vi "VIQA VI Info.vi"(8 "error in (no error)":errorcluster, 10 "Item ID":string, 11 "Project":refnum<vi>) -> (0 "error out":errorcluster, 1 "Valid?":bool, 2 "VI Info":T1, 3 "VI Refnum":refnum<vi>)   [LabVIEW 2018, in "VI Quality.lvlib"]
doc: "This returns VI information about the project item selected."
uses:
  VI Quality.lvlib
  <vilib>/LabVIEW Icon API/LabVIEW Icon API.lvlib
  <vilib>/LabVIEW Icon API/lv_icon/Classes/Icon/Icon.lvclass
  Controls/VIQA VI Info.ctl
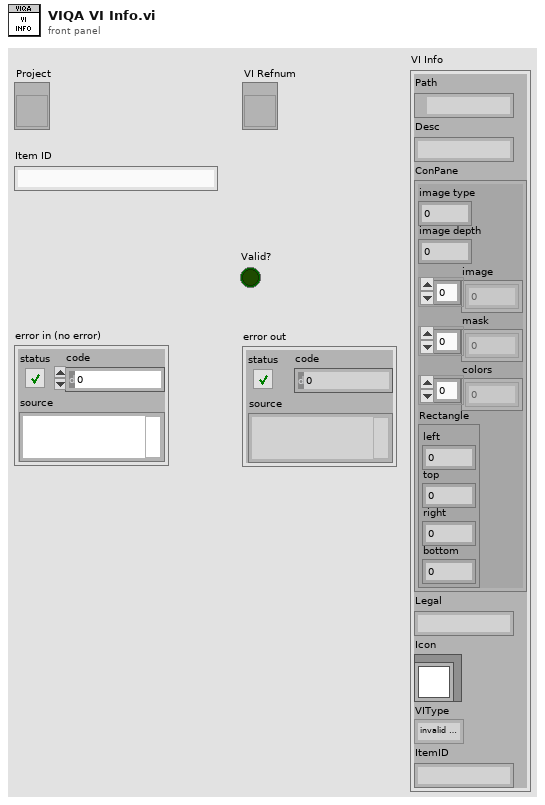
[diagram p1: front panel]
types:
  T1 = typedef "VI Quality.lvlib/VIQA VI Info.ctl" = cluster{"Path":path, "Desc":string, "ConPane":cluster{"image type":i32, "image depth":i32, "image":u8[], "mask":u8[], "colors":u32[], "Rectangle":cluster{"left":i16, "top":i16, "right":i16, "bottom":i16}}, "Legal":string, "Icon":refnum<class "Icon.lvclass">, "VIType":enum32{"invalid VI type", "Standard VI", "Control VI", "Global VI", "Polymorphic VI", "Configuration VI", "SubSystem", "Facade VI", "Method VI", "Statechart Diagram VI"}, "ItemID":string}
  T2 = enum32{"invalid VI type", "Standard VI", "Control VI", "Global VI", "Polymorphic VI", "Configuration VI", "SubSystem", "Facade VI", "Method VI", "Statechart Diagram VI"}
  T3 = typedef "imagedata.ctl" = cluster{"image type":i32, "image depth":i32, "image":u8[], "mask":u8[], "colors":u32[], "Rectangle":cluster{"left":i16, "top":i16, "right":i16, "bottom":i16}}
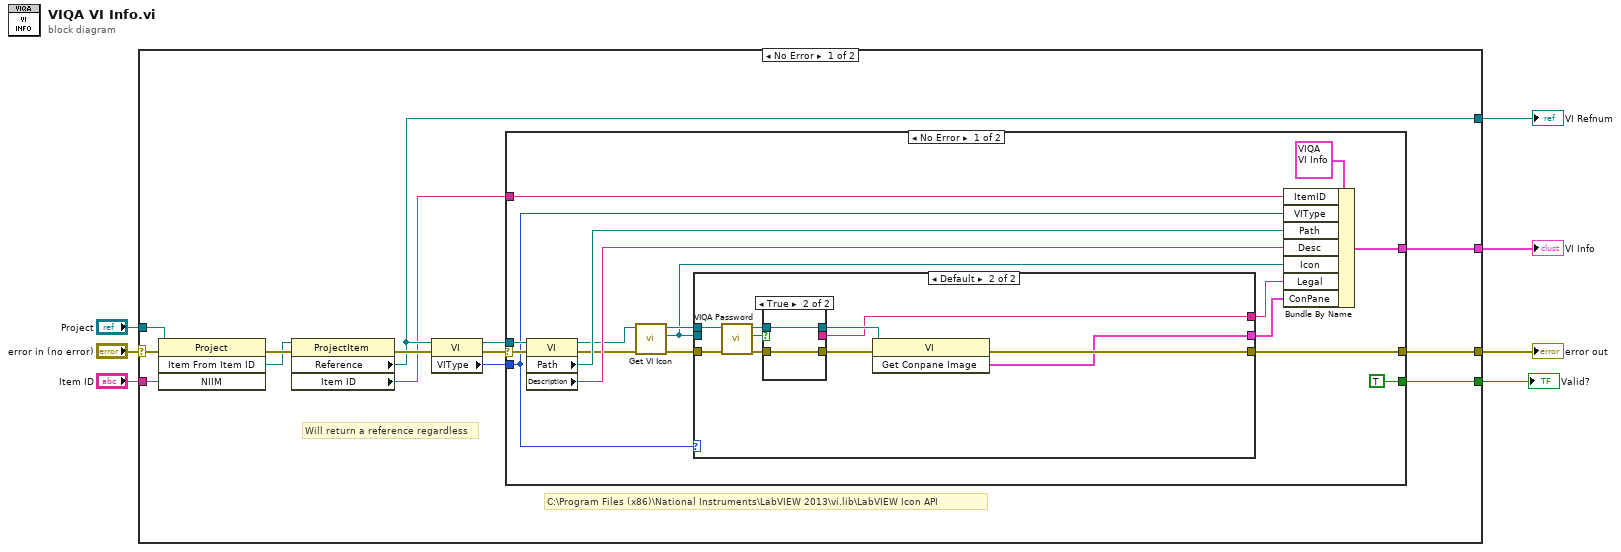
[diagram p0: block diagram]
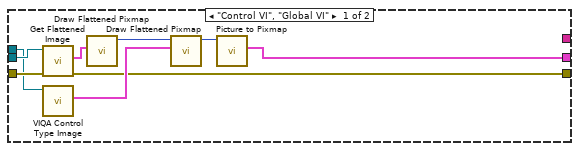
[diagram p2: hidden frame]
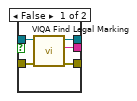
[diagram p3: hidden frame]
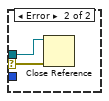
[diagram p4: hidden frame]
diagram:
  n1 = case shown="No Error" "error in (no error)" {
    selector: "error in (no error)" -> [w19 w67]
    tunnel: "Item ID" -> [w18 _]
    tunnel: "Project" -> [w17 _]
    tunnel: [w15 w67] -> w4
    tunnel: [w14 _] -> w3
    tunnel: [w13 _] -> w2
    tunnel: [w9 _] -> w1
    frame No Error {
      # "C:\\Program Files (x86)\\National Instruments\\LabVIEW 2013\\vi.lib\\LabVIEW Icon API"
      # "Will return a reference regardless"
      n2 = invoke class="Project" method="Item From Item ID"(reference=w17, error in=w19, "NIIM"=w18) -> (error out=w21:errorcluster, "GetItemFromNIIM"=w20:refnum<vi>)  [unwired: 1 in, 2 out]
      n3 = property class="ProjectItem"(reference=w20, error in=w21) -> (error out=w16:errorcluster, "Reference"=w13:refnum<vi>, "Item ID"=w8:string)  [unwired: 1 out]
      n4 = property class="VI"(reference=w13, error in=w16) -> (reference out=w12:refnum<vi>, error out=w11:errorcluster, "VIType"=w10:T2)
      n5 = case shown="No Error" w11 {
        selector: w11 -> [w32 w66]
        tunnel: [w38 _] -> w15
        tunnel: [w37 _] -> w14
        tunnel: w12 -> [w33 w65]
        tunnel: w10 -> [w23 _]
        tunnel: [TRUE _] -> w9
        tunnel: w8 -> [w22 _]
        frame No Error {
          n6 = property class="VI"(reference=w33, error in=w32) -> (reference out=w26:refnum<vi>, error out=w31:errorcluster, "Path"=w36:path, "Description"=w35:string)
          n7 = call <vilib>:"Get VI Icon.vi"("error in (no error)"=w31, "VI Refnum in"=w26) -> ("error out"=w30:errorcluster, "Icon"=w28:refnum<class "Icon.lvclass">, "VI Refnum out"=w29:refnum<vi>)  [unwired: 7 in]
          n8 = case shown="Default" w23 {
            tunnel: [w41 w57] -> w38
            tunnel: w30 -> [w47 w52]
            tunnel: w29 -> [w45 w50]
            tunnel: [w39 w56] -> w34
            tunnel: w28 -> [w46 _]
            tunnel: [_ w53] -> w24
            frame "Control VI", "Global VI" {
              n9 = call <vilib>:"Get Flattened Image.vi"("error in (no error)"=w47, "lv_icon.lvlib:Icon.lvclass in"=w46) -> ("error out"=w41:errorcluster, "Color Image"=w44:T3)  [unwired: 6 in, 2 out]
              n10 = call "VIQA Control Type Image.vi"("VI Refnum"=w45) -> ("Type Image"=w43:T3)  [unwired: 8 in, 2 out]
              n11 = call <vilib>:"Draw Flattened Pixmap.vi"("image data"=w44) -> ("new picture"=w42:picture)  [unwired: 8 in]
              n12 = call <vilib>:"Draw Flattened Pixmap.vi"("image data"=w43, "picture"=w42) -> ("new picture"=w40:picture)  [unwired: 7 in]
              n13 = call <vilib>:"Picture to Pixmap.vi"("picture"=w40) -> ("image data"=w39:T3)  [unwired: 9 in, 1 out]
            }
            frame Default {
              n14 = call "VIQA Password.vi"("error in (no error)"=w52, "VI Refnum"=w50) -> ("error out"=w51:errorcluster, "Locked"=w48:bool, "dup VI Refnum"=w49:refnum<vi>)  [unwired: 6 in, 1 out]
              n15 = case shown="True" w48 {
                tunnel: [w62 w63] -> w55
                tunnel: [w61 w64] -> w54
                tunnel: [w60 _] -> w53
                tunnel: w51 -> [w59 w63]
                tunnel: w49 -> [w58 w64]
                frame False {
                  n16 = call "VIQA Find Legal Marking.vi"("error in (no error)"=w59, "VI Refnum"=w58) -> ("error out"=w62:errorcluster, "Legal Marking"=w60:string, "dup VI Refnum"=w61:refnum<vi>)  [unwired: 4 in, 3 out]
                }
                frame True {
                }
              }
              n17 = invoke class="VI" method="Get Conpane Image"(reference=w54, error in=w55) -> (error out=w57:errorcluster, "Get Conpane Image"=w56:T3)  [unwired: 1 in, 1 out]
            }
          }
          n18 = Bundle By Name(cluster=T1 {"Path"=path "", "Desc"="", "ConPane"={"image type"=0, "image depth"=0, "image"=[], "mask"=[], "colors"=[], "Rectangle"={"left"=0, "top"=0, "right"=0, "bottom"=0}}, "Legal"="", "Icon"=refnum, "VIType"=enum."invalid VI type", "ItemID"=""} ("VI Info 2"), "ItemID"=w22, "VIType"=w23, "Path"=w36, "Desc"=w35, "Icon"=w28, "Legal"=w24, "ConPane"=w34) -> (w37:T1)
        }
        frame Error {
          n19 = Close Reference(reference=w65, error in (no error)=w66) -> ()  [unwired: 1 out]
        }
      }
    }
    frame Error {
    }
  }
  "error out" <- w4
  "VI Info" <- w3
  "VI Refnum" <- w2
  "Valid?" <- w1
